vi "main.vi"() -> ()   [LabVIEW 2012]
doc: "Game of Life\nDefines an environment (occupancy grid) containing a robot and food squares. The robot aims to search out food squares such that it will live as long as possible."
panel:
  out "Step":i32
  out "Energy":i8(slide) scale=0.0..30.0
  in  "Cycle Delay":u32(slide) step=25 scale=50.0..2000.0
  out "V_Heading":i8
  out "Sense Heading":i8
  in  "Food per level":i32
  in  "Level":i32
  out "Y":i8
  out "X":i8
  in  "estop":bool
  out "Heartbeat":bool
  in  "Tab Control":enum32{"Initial World Data", "World Graph"}(tab)
  out "Initial World":i8[][](graph)
  out "World":i8[][](graph)
  # "Robot Position"
  # "Difficulty"
  # "V Code\n  6 7 8\n  5 0 1\n  4 3 2"
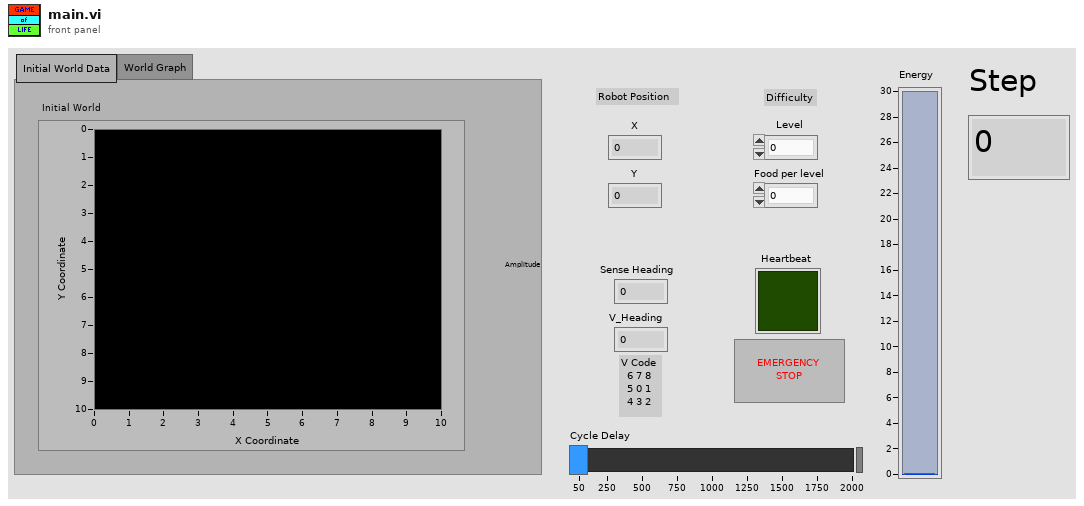
[diagram p1: front panel]
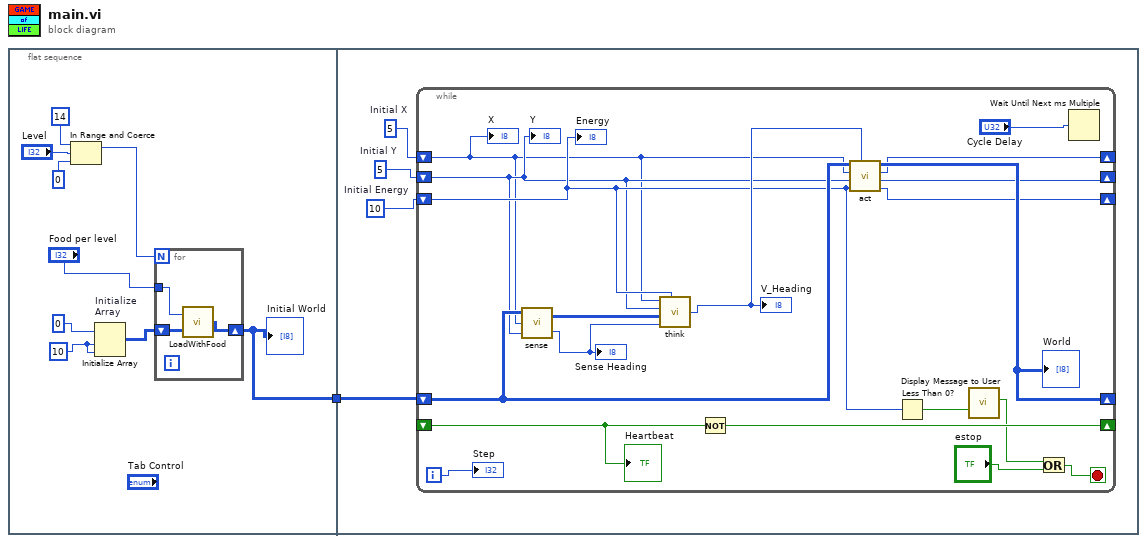
[diagram p0: block diagram]
diagram:
  n1 = flat-sequence {
    tunnel: [w2] -> w1
    tunnel: w1 -> [w17]
    frame #0 {
      w9 = 10
      n2 = In Range and Coerce(upper limit=14, x="Level", lower limit=0) -> (coerced(x)=w5:i32)  [unwired: 1 out]
      n3 = Initialize Array "Initialize \nArray"(i8 0, w9, w9) -> (w3:i8[][])
      n4 = for {
        N: w5 -> [_]
        tunnel: "Food per level" -> [w13]
        shift-right: [w11] -> w2
        shift-left: w3 -> [w12]
        n5 = call "LoadWithFood.vi"("Input Array"=w12, "Food Per Level"=w13) -> ("Output Array"=w11:i8[][])
      }
      "Initial World" <- w2
    }
    frame #1 {
      w14 = i8 10  # Initial Energy
      w16 = i8 5  # Initial Y
      w15 = i8 5  # Initial X
      n6 = while {
        shift-right: [w35] -> _
        shift-left: _ -> [w36]
        shift-right: [w33] -> _
        shift-left: w17 -> [w29]
        shift-right: [w32] -> _
        shift-left: w15 -> [w19]
        shift-right: [w31] -> _
        shift-left: w16 -> [w20]
        shift-right: [w30] -> _
        shift-left: w14 -> [w23]
        i -> [w18]
        stop <- w28 stop-if-true
        n7 = call "sense.vi"("Y"=w20, "X"=w19, "World"=w29) -> ("Heading"=w22:i8, "Sensor Array"=w21:i8[][])
        "Sense Heading" <- w22
        n8 = call "think.vi"("X"=w19, "Y"=w20, "Sensor Array"=w21, "Sense Heading"=w22, "E"=w23) -> ("V Heading"=w24:i8)
        "V_Heading" <- w24
        n9 = Not(x=w36) -> (.not. x?=w35:bool)
        n10 = call "act.vi"("V"=w24, "Ein"=w23, "Yin"=w20, "Xin"=w19, "Input Array"=w29) -> ("Eout"=w30:i8, "Yout"=w31:i8, "Xout"=w32:i8, "Output Array"=w33:i8[][])
        "World" <- w33
        n11 = Less Than 0?(x=w23) -> (x < 0?=w25:bool)
        n12 = call "Display Message to User"("Enable"=w25) -> ("Quit"=w26:bool)  [unwired: 9 in, 1 out]
        n13 = Or(x=w26, y="estop") -> (x .or. y?=w28:bool)
        n14 = Wait Until Next ms Multiple(millisecond multiple="Cycle Delay") -> ()  [unwired: 1 out]
        "X" <- w19
        "Energy" <- w23
        "Y" <- w20
        "Heartbeat" <- w36
        "Step" <- w18
      }
    }
  }
